vi "MakeXyData.vi"(8 "error in (no error)":errorcluster caption="エラー入力（エラーなし）", 10 "時間列(1～) ref":refnum<vi>, 11 "表 ref":refnum<vi>) -> (0 "error out":errorcluster caption="エラー出力")   [LabVIEW 2014]
uses:
  GlobalData/GlobalXyData.vi
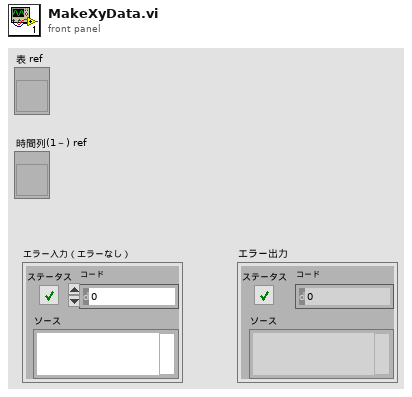
[diagram p1: front panel]
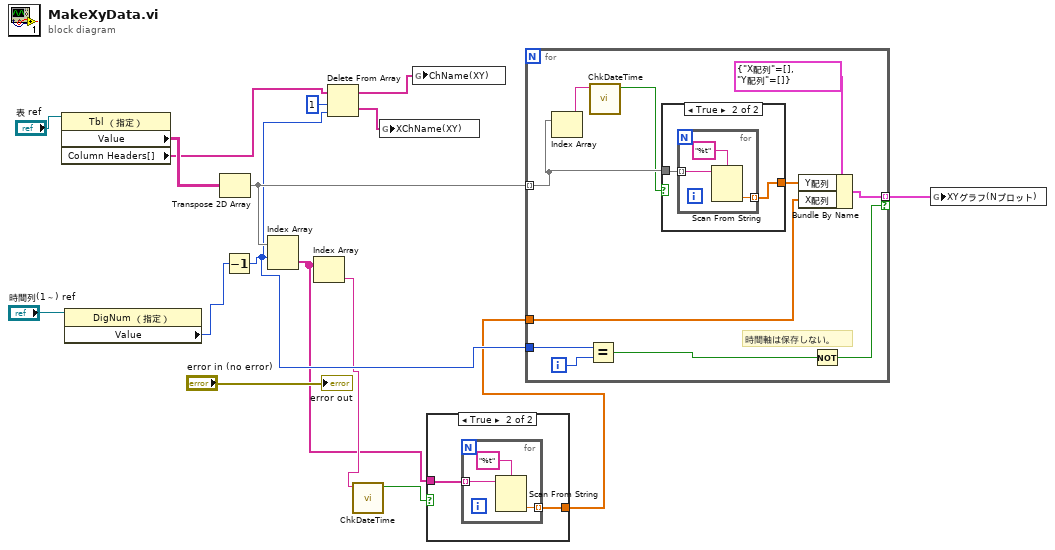
[diagram p0: block diagram]
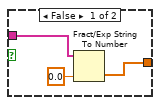
[diagram p2: hidden frame]
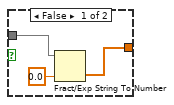
[diagram p3: hidden frame]
diagram:
  n1 = property class="Tbl （指定）"(reference="表 ref") -> ("Value"=w14:string[][], "Column Headers[]"=w9:string[])  [unwired: 1 in, 2 out]
  n2 = property class="DigNum （指定）"(reference="時間列(1～) ref") -> ("Value"=w12:i32)  [unwired: 1 in, 2 out]
  n3 = Transpose 2D Array(2D array=w14) -> (transposed array=w11:string[][])
  n4 = Decrement(x=w12) -> (x-1=w8:i32)
  n5 = Index Array(array=w11, index (row)=w8) -> (element=w3:string[])  [unwired: 1 in]
  n6 = Index Array(array=w3) -> (element=w4:string)  [unwired: 1 in]
  n7 = Delete From Array(array=w9, length=1 ("長さ"), index=w8) -> (deleted portion=w6:string[], array with subset deleted=w7:string[])
  n8 = call "ChkDateTime.vi"("文字列"=w4) -> ("ブール"=w5:bool)  [unwired: 10 in]
  n9 = global write "GlobalXyData.vi" "XChName(XY)"(w6) -> ()
  n10 = global write "GlobalXyData.vi" "ChName(XY)"(w7) -> ()
  n11 = case shown="TRUE" w5 {
    tunnel: w3 -> [w18 w21]
    tunnel: [w17 w20] -> w2
    frame False {
      n12 = Fract/Exp String To Number(string=w18, default (0 dbl)=0.0 ("デフォルト（0 I32）")) -> (number=w17:dbl[])  [unwired: 2 in, 1 out]
    }
    frame True {
      n13 = for {
        tunnel: w21 -> [w23] mode=indexing
        tunnel: [w22] -> w20 mode=indexing
        n14 = Scan From String(format string="%t" ("形式文字列"), input string=w23) -> (output 1=w22:dbl)  [unwired: 3 in, 3 out]
      }
    }
  }
  n15 = for {
    tunnel: w8 -> [w34]
    tunnel: w11 -> [w27] mode=indexing
    tunnel: w2 -> [w29]
    tunnel: [w31] -> w1 mode=indexing if=w30
    i -> [w35]
    # "時間軸は保存しない。"
    n16 = Index Array(array=w27) -> (element=w26:string)  [unwired: 1 in]
    n17 = Equal?(x=w34, y=w35) -> (x = y?=w33:bool)
    n18 = call "ChkDateTime.vi"("文字列"=w26) -> ("ブール"=w25:bool)  [unwired: 10 in]
    n19 = case shown="TRUE" w25 {
      tunnel: w27 -> [w37 w40]
      tunnel: [w36 w39] -> w28
      frame False {
        n20 = Fract/Exp String To Number(string=w37, default (0 dbl)=0.0 ("デフォルト（0 I32）")) -> (number=w36:dbl[])  [unwired: 2 in, 1 out]
      }
      frame True {
        n21 = for {
          tunnel: w40 -> [w42] mode=indexing
          tunnel: [w41] -> w39 mode=indexing
          n22 = Scan From String(format string="%t" ("形式文字列"), input string=w42) -> (output 1=w41:dbl)  [unwired: 3 in, 3 out]
        }
      }
    }
    n23 = Bundle By Name(cluster=cluster{"X配列":dbl[], "Y配列":dbl[]} {"X配列"=[], "Y配列"=[]} ("クラスタ"), "Y配列"=w28, "X配列"=w29) -> (w31:cluster{"X配列":dbl[], "Y配列":dbl[]})
    n24 = Not(x=w33) -> (.not. x?=w30:bool)
  }
  n25 = global write "GlobalXyData.vi" "XYグラフ(Nプロット)"(w1) -> ()
  "error out" <- "error in (no error)"
